vi "Read User Info.vi"(8 "error in (no error)":errorcluster, 11 "mqtt in":refnum<class "mqtt.lvclass">) -> (0 "error out":errorcluster, 2 "User Info":T1={"User Name"="User", "Password"="password"}, 3 "mqtt out":refnum<class "mqtt.lvclass">)   [LabVIEW 2020, in "mqtt.lvclass"]
uses:
  mqtt.lvclass
  mqttTypedef/mqttUserInfo.ctl
  mqtt.lvclass/mqtt.ctl
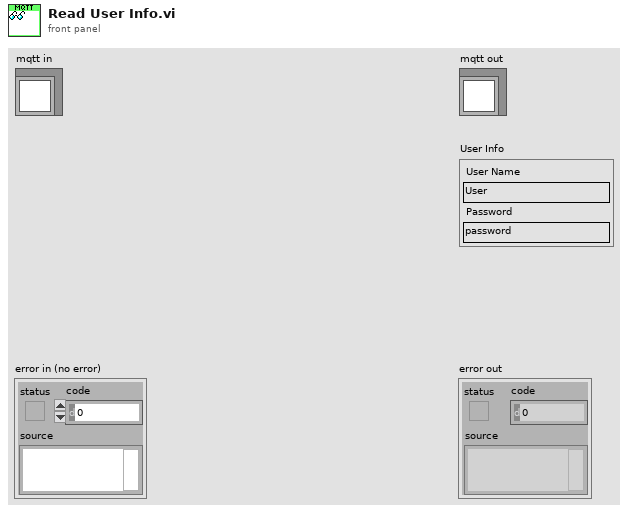
[diagram p1: front panel]
types:
  T1 = typedef "mqtt.lvclass/mqttUserInfo.ctl" = cluster{"User Name":string, "Password":string}
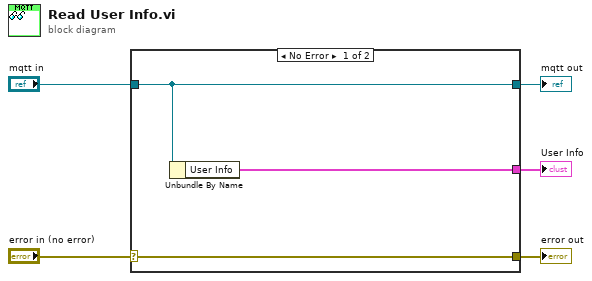
[diagram p0: block diagram]
diagram:
  n1 = case shown="No Error" "error in (no error)" {
    selector: "error in (no error)" -> [w8 w9]
    tunnel: [w8 w9] -> w4
    tunnel: [w7 w10] -> w2
    tunnel: "mqtt in" -> [w7 w10]
    tunnel: [w6 _] -> w1
    frame No Error {
      n2 = Unbundle By Name(w7) -> ("User Info"=w6:T1)
    }
    frame Error {
    }
  }
  "error out" <- w4
  "mqtt out" <- w2
  "User Info" <- w1
